vi "_PC_Daemon setParamSampleType.vi"() -> ()   [LabVIEW 2018]
uses:
  <vilib>/Utility/file.llb/Read Delimited Spreadsheet (string).vi
  <vilib>/Utility/file.llb/Write Delimited Spreadsheet (string).vi
panel:
  in  "sampleTypeTable":string[][](table)=[["", ""], ["", ""], ["", ""]]
  in  "exit":bool
  in  "saveAsData":bool caption="saveas_data"
  in  "saveData":bool caption="save_data"
  in  "loadData":bool caption="load_data"
  out "checkRow":i32
  out "error out":errorcluster
  in  "error in (no error)":errorcluster
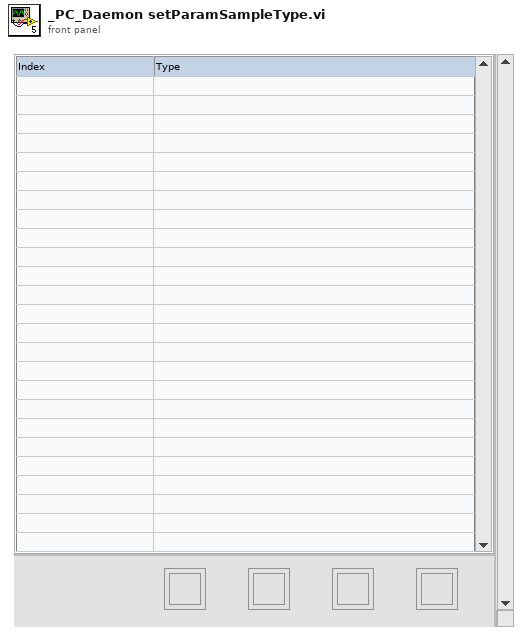
[diagram p1: front panel]
types:
  T1 = typedef "LVPoint32TypeDef.ctl" = cluster{"Horizontal":i32, "Vertical":i32}
  T2 = typedef "LVRowAndColumnTypeDef.ctl" = cluster{"Row":i32, "Column":i32}
  T3 = typedef "eventvkey.ctl" = enum16{"ASCII", "Enter", "Return", "Shift", "Ctrl", "Alt", "Cmd", "Opt", "Caps", "NumLock", "Clear", "Break", "Up", "Down", "Left", "Right", "Insert", "Delete", "Home", "End", "PageUp", "PageDown", "Escape", "Help", "Pause", "ScrollLock", "F1", "F2", "F3", "F4", "F5", "F6", "F7", "F8", "F9", "F10", "F11", "F12", "F13", "F14", "F15", "F16", "F17", "F18", "F19", "F20", "F21", "F22", "F23", "F24", "Play", "VolumeUp", "VolumeDown", "Mute", "Two Byte Char"}
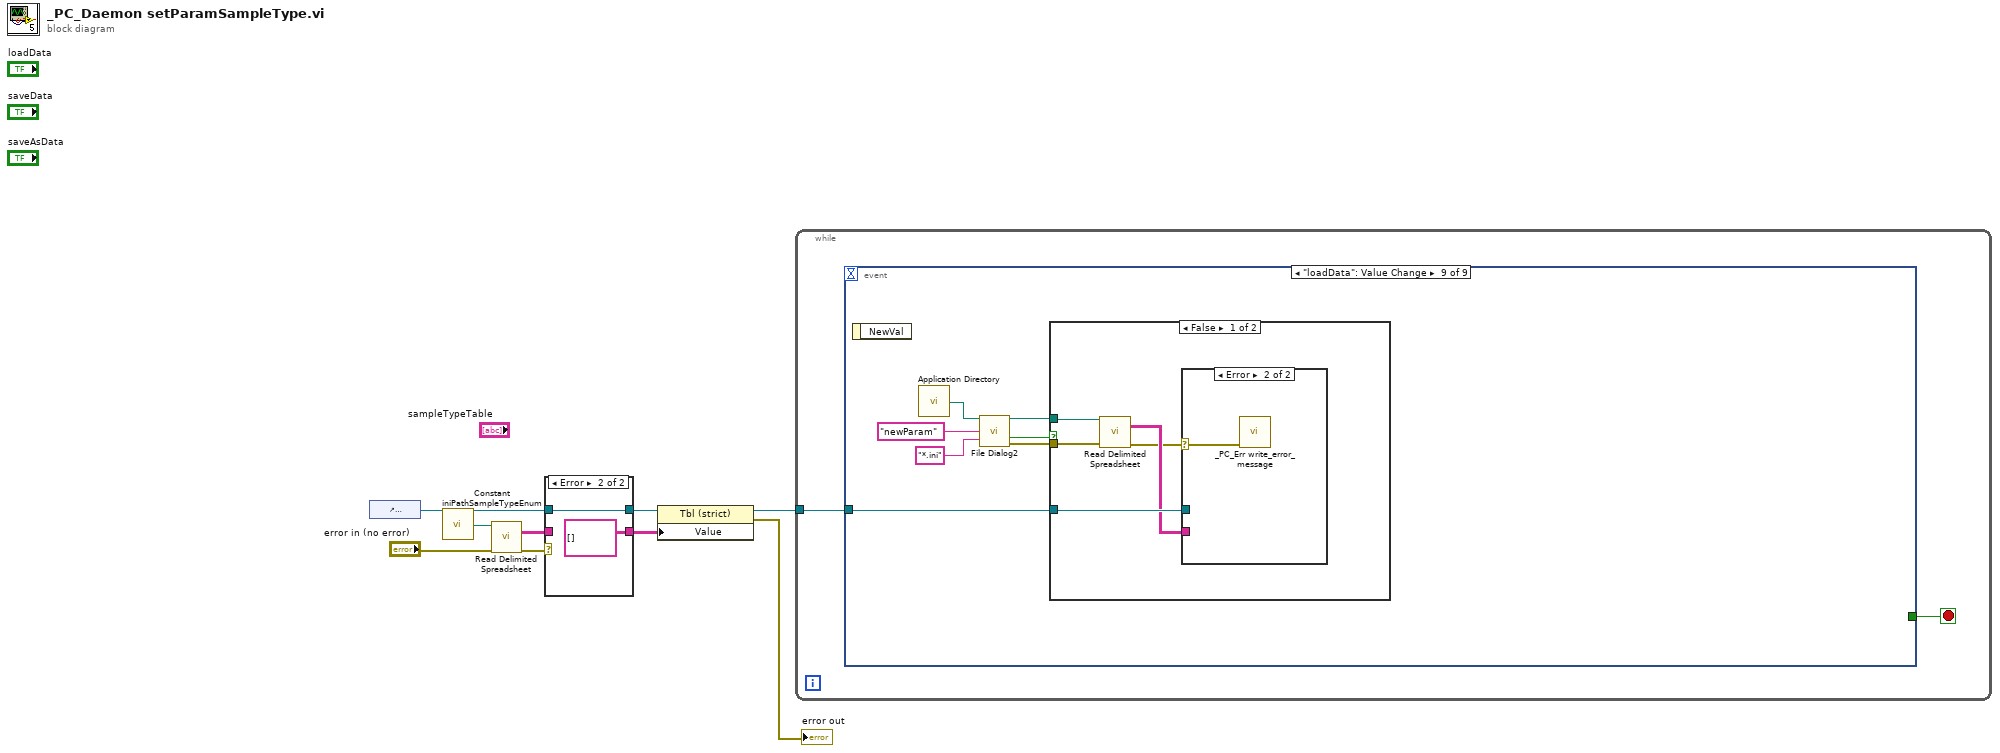
[diagram p0: block diagram]
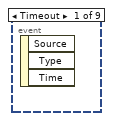
[diagram p3: hidden frame]
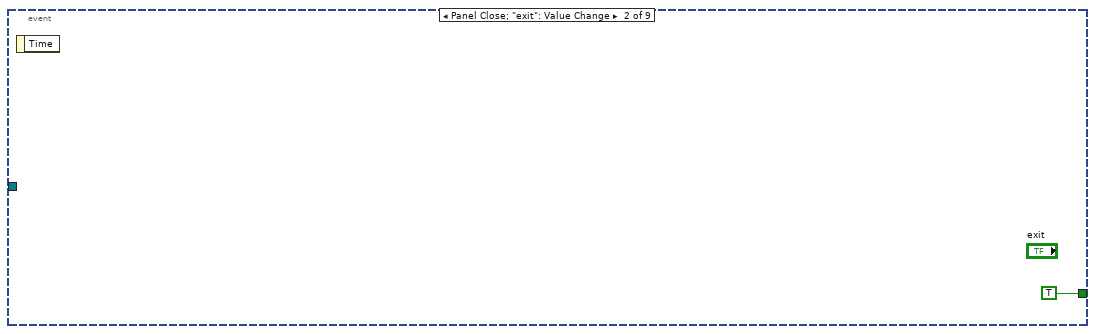
[diagram p4: hidden frame]
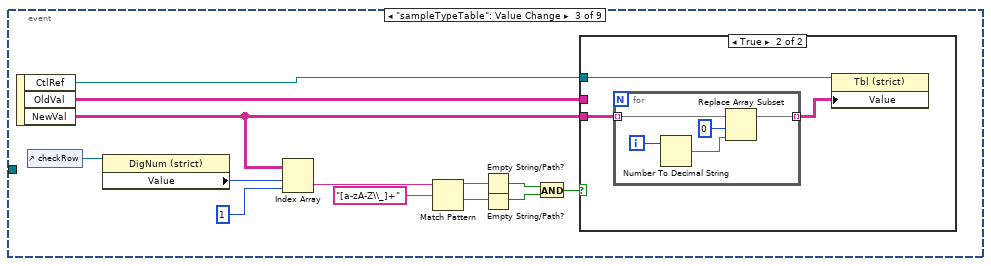
[diagram p5: hidden frame]
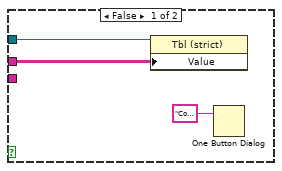
[diagram p6: hidden frame]
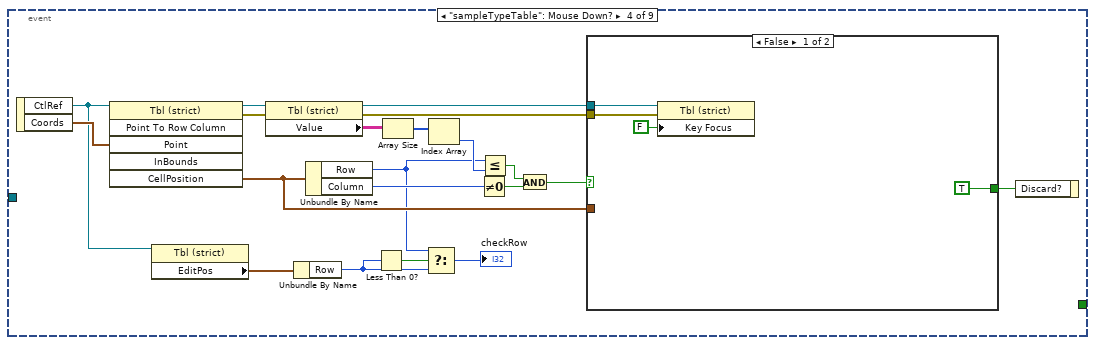
[diagram p7: hidden frame]
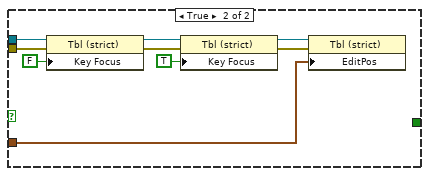
[diagram p8: hidden frame]
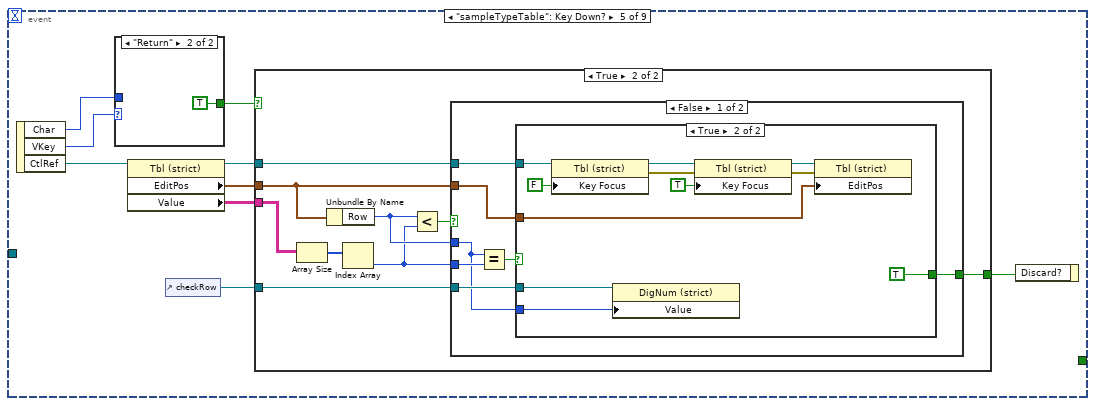
[diagram p9: hidden frame]
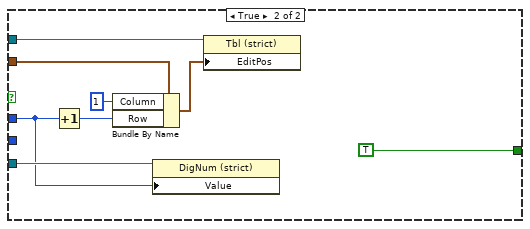
[diagram p12: hidden frame]
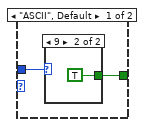
[diagram p13: hidden frame]
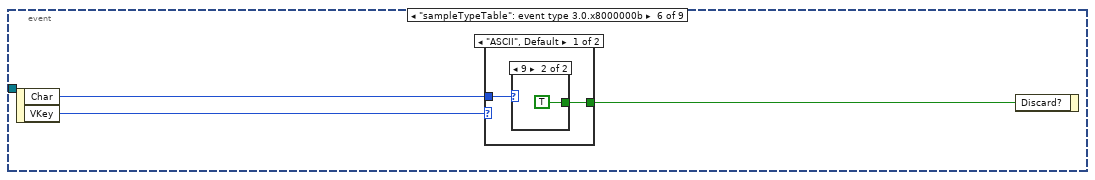
[diagram p15: hidden frame]
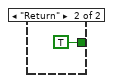
[diagram p17: hidden frame]
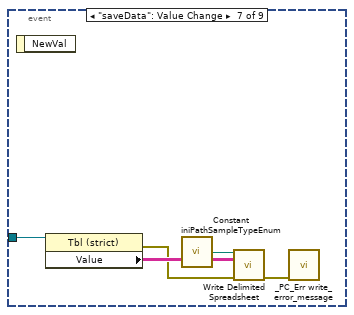
[diagram p18: hidden frame]
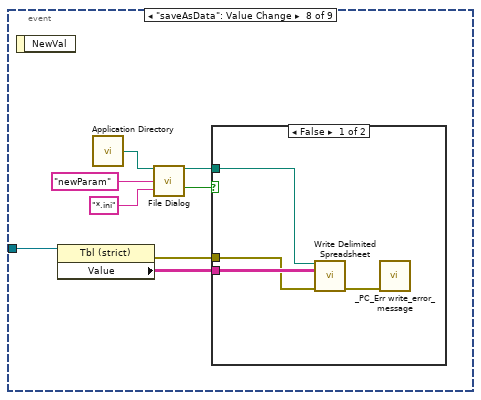
[diagram p19: hidden frame]
diagram:
  n1 = control-ref of="sampleTypeTable"() -> (w9:refnum<vi>)
  n2 = call "Constant iniPathSampleTypeEnum.vi"() -> ("appended path"=w8:path)
  n3 = call-poly <vilib>:"Read Delimited Spreadsheet.vi"("file path (dialog if empty)"=w8, "error in (no error)"="error in (no error)") -> ("all rows"=w6:string[][], "error out"=w5:errorcluster)  [unwired: 8 in, 4 out]
  n4 = case shown="Error" w5 {
    tunnel: w9 -> [w11 w13]
    tunnel: [w11 w13] -> w4
    tunnel: w6 -> [w10 _]
    tunnel: [w10 string[][] [] ("all rows")] -> w3
    frame No Error {
    }
    frame Error {
    }
  }
  n5 = property class="Tbl (strict)"(reference=w4, "Value"=w3) -> (reference out=w2:refnum<vi>, error out=→"error out":errorcluster)  [unwired: 1 in]
  n6 = while {
    tunnel: w2 -> [w14]
    stop <- w15 stop-if-true
    n7 = event shown="[8] \"loadData\": Value Change" {
      selector: _ -> [_ _ _ _ _ _ _ _ _]
      dyn-events: _ -> [_ _ _ _ _ _ _ _ _]
      timeout: _ -> [_ _ _ _ _ _ _ _ _]
      tunnel: [_ TRUE _ _ _ _ _ _ _] -> w15
      tunnel: w14 -> [_ _ _ _ _ _ w133 w139 w147]
      event Timeout {
        n8 = event-data() -> ()  [unwired: 1 in, 3 out]
      }
      event Panel Close; "exit": Value Change {
        n9 = event-data() -> ()  [unwired: 1 in, 1 out]
      }
      event "sampleTypeTable": Value Change {
        n10 = event-data() -> ("CtlRef"=w24:refnum<vi>, "OldVal"=w21:string[][], "NewVal"=w17:string[][])  [unwired: 1 in]
        n11 = control-ref of="checkRow"() -> (w29:refnum<vi>)
        n12 = property class="DigNum (strict)"(reference=w29) -> ("Value"=w28:i32)  [unwired: 1 in, 2 out]
        n13 = Index Array(array=w17, index (row)=w28, index (col)=1 ("disabled index (col)")) -> (element=w26:string)
        n14 = Match Pattern(string=w26, regular expression="[a-zA-Z\\_]+") -> (before substring=w23:string, after substring=w22:string)  [unwired: 1 in, 2 out]
        n15 = Empty String/Path?(string/path=w23) -> (empty?=w20:bool)
        n16 = Empty String/Path?(string/path=w22) -> (empty?=w19:bool)
        n17 = And(x=w20, y=w19) -> (x .and. y?=w18:bool)
        n18 = case shown="True" w18 {
          tunnel: w24 -> [w32 w34]
          tunnel: w21 -> [w31 _]
          tunnel: w17 -> [_ w35]
          frame False {
            n19 = property class="Tbl (strict)"(reference=w32, "Value"=w31) -> ()  [unwired: 1 in, 2 out]
            n20 = One Button Dialog(message="Contains incorrect characters") -> ()  [unwired: 1 in, 1 out]
          }
          frame True {
            n21 = for {
              tunnel: w35 -> [w40] mode=indexing
              tunnel: [w36] -> w33 mode=indexing
              i -> [w38]
              n22 = Number To Decimal String(number=w38) -> (decimal integer string=w37:string)  [unwired: 1 in]
              n23 = Replace Array Subset(array=w40, new element=w37, index=0) -> (w36:string[])
            }
            n24 = property class="Tbl (strict)"(reference=w34, "Value"=w33) -> ()  [unwired: 1 in, 2 out]
          }
        }
      }
      event "sampleTypeTable": Mouse Down? {
        n25 = event-data() -> ("CtlRef"=w46:refnum<vi>, "Coords"=w60:T1)  [unwired: 1 in]
        n26 = invoke class="Tbl (strict)" method="Point To Row Column"(reference=w46, "Point"=w60) -> (reference out=w59:refnum<vi>, error out=w58:errorcluster, "CellPosition"=w47:T2)  [unwired: 4 in, 3 out]
        n27 = property class="Tbl (strict)"(reference=w46) -> ("EditPos"=w45:T2)  [unwired: 1 in, 2 out]
        n28 = property class="Tbl (strict)"(reference=w59, error in=w58) -> (reference out=w50:refnum<vi>, error out=w49:errorcluster, "Value"=w57:string[][])
        n29 = Unbundle By Name(w45) -> ("Row"=w42:i32)
        n30 = Unbundle By Name(w47) -> ("Row"=w43:i32, "Column"=w55:i32)
        n31 = Less Than 0?(x=w42) -> (x < 0?=w44:bool)
        n32 = Array Size(array=w57) -> (size(s)=w56:i32[])
        n33 = Select(t=w43, s=w44, f=w42) -> (s? t:f=→"checkRow":i32)
        n34 = Index Array(array=w56) -> (element=w48:i32)  [unwired: 1 in]
        n35 = Not Equal To 0?(x=w55) -> (x != 0?=w53:bool)
        n36 = Less Or Equal?(x=w43, y=w48) -> (x <= y?=w54:bool)
        n37 = And(x=w54, y=w53) -> (x .and. y?=w52:bool)
        n38 = case shown="False" w52 {
          tunnel: [TRUE _] -> w51
          tunnel: w50 -> [w63 w73]
          tunnel: w49 -> [w62 w72]
          tunnel: w47 -> [_ w65]
          frame False {
            n39 = property class="Tbl (strict)"(reference=w63, error in=w62, "Key Focus"=FALSE) -> ()  [unwired: 2 out]
          }
          frame True {
            n40 = property class="Tbl (strict)"(reference=w73, error in=w72, "Key Focus"=FALSE) -> (reference out=w67:refnum<vi>, error out=w66:errorcluster)
            n41 = property class="Tbl (strict)"(reference=w67, error in=w66, "Key Focus"=TRUE) -> (reference out=w68:refnum<vi>, error out=w69:errorcluster)
            n42 = property class="Tbl (strict)"(reference=w68, error in=w69, "EditPos"=w65) -> ()  [unwired: 2 out]
          }
        }
        n43 = event-data("Discard?"=w51) -> ()  [unwired: 1 in, 1 out]
      }
      event "sampleTypeTable": Key Down? {
        n44 = event-data() -> ("Char"=w81:i16, "VKey"=w82:T3, "CtlRef"=w80:refnum<vi>)  [unwired: 1 in]
        n45 = case shown="\"Return\"" w82 {
          tunnel: w81 -> [w119 _]
          tunnel: [w118 TRUE] -> w79
          frame "ASCII", Default {
            n46 = case shown="9" w119 {
              tunnel: [_ TRUE] -> w118
              frame 0, Default {
              }
              frame 9 {
              }
            }
          }
          frame "Return" {
          }
        }
        n47 = property class="Tbl (strict)"(reference=w80) -> (reference out=w78:refnum<vi>, "EditPos"=w77:T2, "Value"=w76:string[][])  [unwired: 1 in, 1 out]
        n48 = control-ref of="checkRow"() -> (w75:refnum<vi>)
        n49 = case shown="True" w79 {
          tunnel: w78 -> [_ w88]
          tunnel: w77 -> [_ w87]
          tunnel: w76 -> [_ w90]
          tunnel: w75 -> [_ w86]
          tunnel: [_ w84] -> w74
          frame False {
          }
          frame True {
            n50 = Array Size(array=w90) -> (size(s)=w91:i32[])
            n51 = Unbundle By Name(w87) -> ("Row"=w85:i32)
            n52 = Index Array(array=w91) -> (element=w83:i32)  [unwired: 1 in]
            n53 = Less?(x=w85, y=w83) -> (x < y?=w89:bool)
            n54 = case shown="False" w89 {
              tunnel: w88 -> [w96 w117]
              tunnel: w87 -> [w94 w116]
              tunnel: w85 -> [w92 w110]
              tunnel: w86 -> [w93 w113]
              tunnel: [w95 TRUE] -> w84
              tunnel: w83 -> [w98 _]
              frame False {
                n55 = Equal?(x=w92, y=w98) -> (x = y?=w97:bool)
                n56 = case shown="True" w97 {
                  tunnel: w96 -> [_ w109]
                  tunnel: [_ TRUE] -> w95
                  tunnel: w94 -> [_ w102]
                  tunnel: w93 -> [_ w100]
                  tunnel: w92 -> [_ w99]
                  frame False {
                  }
                  frame True {
                    n57 = property class="Tbl (strict)"(reference=w109, "Key Focus"=FALSE) -> (reference out=w107:refnum<vi>, error out=w106:errorcluster)  [unwired: 1 in]
                    n58 = property class="DigNum (strict)"(reference=w100, "Value"=w99) -> ()  [unwired: 1 in, 2 out]
                    n59 = property class="Tbl (strict)"(reference=w107, error in=w106, "Key Focus"=TRUE) -> (reference out=w101:refnum<vi>, error out=w103:errorcluster)
                    n60 = property class="Tbl (strict)"(reference=w101, error in=w103, "EditPos"=w102) -> ()  [unwired: 2 out]
                  }
                }
              }
              frame True {
                n61 = Increment(x=w110) -> (x+1=w111:i32)
                n62 = Bundle By Name(cluster=w116, "Column"=1, "Row"=w111) -> (w115:T2)
                n63 = property class="DigNum (strict)"(reference=w113, "Value"=w110) -> ()  [unwired: 1 in, 2 out]
                n64 = property class="Tbl (strict)"(reference=w117, "EditPos"=w115) -> ()  [unwired: 1 in, 2 out]
              }
            }
          }
        }
        n65 = event-data("Discard?"=w74) -> ()  [unwired: 1 in, 1 out]
      }
      event "sampleTypeTable": event type 3.0.x8000000b {
        n66 = event-data() -> ("Char"=w123:i16, "VKey"=w124:T3)  [unwired: 1 in]
        n67 = case shown="\"ASCII\", Default" w124 {
          tunnel: w123 -> [w126 _]
          tunnel: [w125 TRUE] -> w122
          frame "ASCII", Default {
            n68 = case shown="9" w126 {
              tunnel: [_ TRUE] -> w125
              frame 0, Default {
              }
              frame 9 {
              }
            }
          }
          frame "Return" {
          }
        }
        n69 = event-data("Discard?"=w122) -> ()  [unwired: 1 in, 1 out]
      }
      event "saveData": Value Change {
        n70 = event-data() -> ()  [unwired: 1 in, 1 out]
        n71 = property class="Tbl (strict)"(reference=w133) -> (error out=w130:errorcluster, "Value"=w131:string[][])  [unwired: 1 in, 1 out]
        n72 = call "Constant iniPathSampleTypeEnum.vi"() -> ("appended path"=w132:path)
        n73 = call-poly <vilib>:"Write Delimited Spreadsheet.vi"("file path (dialog if empty)"=w132, "2D data"=w131, "error in (no error)"=w130) -> ("error out"=w129:errorcluster)  [unwired: 11 in, 1 out]
        n74 = call "_PC_Err write_error_message.vi"("error in"=w129) -> ()  [unwired: 10 in, 1 out]
      }
      event "saveAsData": Value Change {
        n75 = event-data() -> ()  [unwired: 1 in, 1 out]
        n76 = property class="Tbl (strict)"(reference=w139) -> (error out=w140:errorcluster, "Value"=w141:string[][])  [unwired: 1 in, 1 out]
        n77 = call <vilib>:"Application Directory.vi"() -> ("Application Directory"=w138:path)
        n78 = call "File Dialog"("start path"=w138, "default name"="newParam", "pattern (all files)"="*.ini") -> ("selected path"=w135:path, "cancelled"=w134:bool)  [unwired: 9 in, 2 out]
        n79 = case shown="False" w134 {
          tunnel: w141 -> [w144 _]
          tunnel: w140 -> [w143 _]
          tunnel: w135 -> [w145 _]
          frame False {
            n80 = call-poly <vilib>:"Write Delimited Spreadsheet.vi"("file path (dialog if empty)"=w145, "2D data"=w144, "error in (no error)"=w143) -> ("error out"=w142:errorcluster)  [unwired: 11 in, 1 out]
            n81 = call "_PC_Err write_error_message.vi"("error in"=w142) -> ()  [unwired: 10 in, 1 out]
          }
          frame True {
          }
        }
      }
      event "loadData": Value Change {
        n82 = event-data() -> ()  [unwired: 1 in, 1 out]
        n83 = call <vilib>:"Application Directory.vi"() -> ("Application Directory"=w152:path)
        n84 = call "File Dialog2"("start path"=w152, "default name"="newParam", "pattern (all files)"="*.ini") -> ("selected path"=w149:path, "cancelled"=w148:bool, "error out"=w146:errorcluster)  [unwired: 9 in, 1 out]
        n85 = case shown="False" w148 {
          tunnel: w149 -> [w156 _]
          tunnel: w147 -> [w157 _]
          tunnel: w146 -> [w155 _]
          frame False {
            n86 = call-poly <vilib>:"Read Delimited Spreadsheet.vi"("file path (dialog if empty)"=w156, "error in (no error)"=w155) -> ("all rows"=w154:string[][], "error out"=w153:errorcluster)  [unwired: 8 in, 4 out]
            n87 = case shown="Error" w153 {
              selector: w153 -> [_ w160]
              tunnel: w157 -> [w159 _]
              tunnel: w154 -> [w158 _]
              frame No Error {
                n88 = property class="Tbl (strict)"(reference=w159, "Value"=w158) -> ()  [unwired: 1 in, 2 out]
              }
              frame Error {
                n89 = call "_PC_Err write_error_message.vi"("error in"=w160) -> ()  [unwired: 10 in, 1 out]
              }
            }
          }
          frame True {
          }
        }
      }
    }
  }
